vi "Main.vi"() -> ()   [LabVIEW 2015]
doc: "Use this template to build a master/slave design pattern. The master loop always executes. It notifies one or more slave loops to execute their code. The slave loop(s) continue executing until they complete, then wait for another notification. Contrast this with the Producer/Consumer pattern in which the consumer loops execute only when they have data in their queue."
uses:
  System SubVIs/Notifier Messages.ctl
panel:
  out "BPM Size":bool
  out "Axis Positions":sgl[](array[numeric])
  in  "Run Scan":bool
  in  "Home Motors":bool
  in  "stop":bool
  # "X1"
  # "Y1"
  # "X2"
  # "Y2"
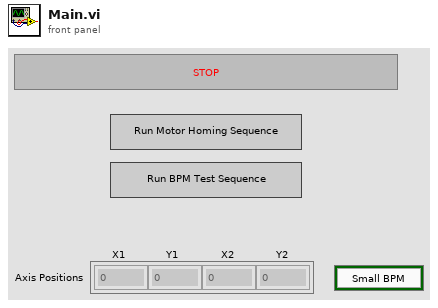
[diagram p1: front panel]
types:
  T1 = typedef "Notifier Messages.ctl" = enum16{"Do Nothing", "Run Scan", "Home Motors"}
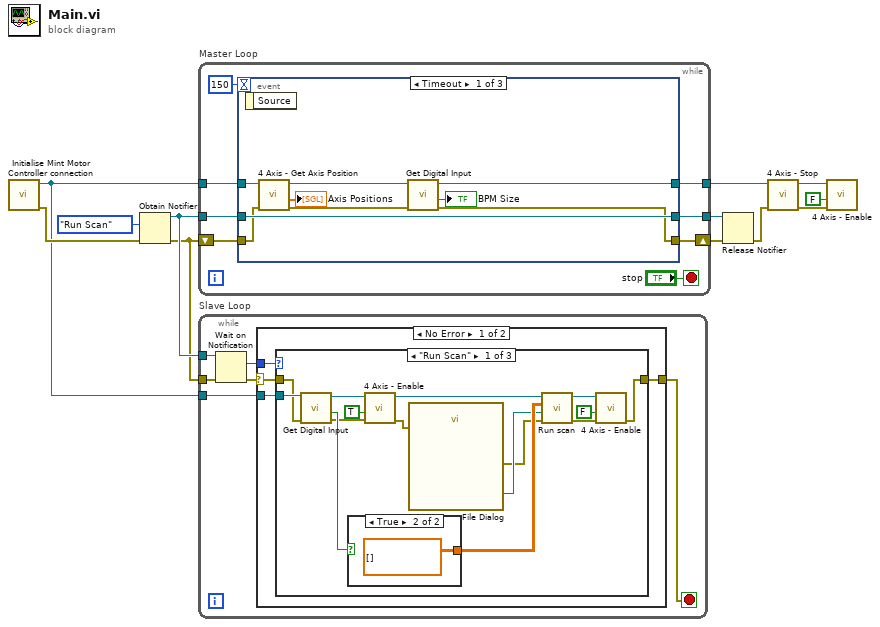
[diagram p0: block diagram]
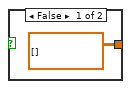
[diagram p2: hidden frame]
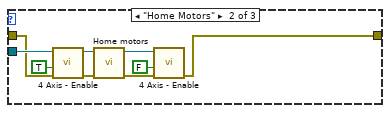
[diagram p3: hidden frame]
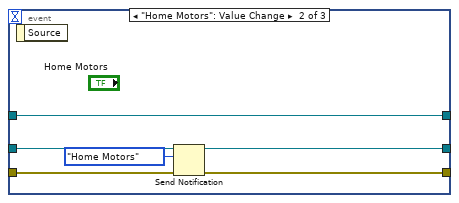
[diagram p6: hidden frame]
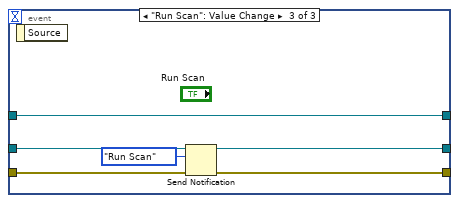
[diagram p7: hidden frame]
diagram:
  n1 = call "Initialise Mint Motor Controller connection.vi"() -> ("error out"=w7:errorcluster, "Controller reference out"=w6:refnum<k7>)  [unwired: 6 in]
  n2 = Obtain Notifier(notification data type=Notifier_Messages."Run Scan", error in (no error)=w7) -> (notifier out=w12:refnum<notifier>, error out=w8:errorcluster)  [unwired: 1 in, 2 out]
  n3 = while "Master Loop" {
    shift-right: [w15] -> w11
    shift-left: w8 -> [w17]
    tunnel: w12 -> [w18]
    tunnel: [w16] -> w10
    tunnel: w6 -> [w14]
    tunnel: [w13] -> w5
    stop <- "stop" stop-if-true
    n4 = event shown="[0] Timeout" {
      selector: _ -> [_ _ _]
      dyn-events: _ -> [_ _ _]
      timeout: 150 -> [_ _ _]
      tunnel: w18 -> [w29 w35 w41]
      tunnel: w17 -> [w27 w34 w40]
      tunnel: [w29 w33 w39] -> w16
      tunnel: [w23 w32 w38] -> w15
      tunnel: w14 -> [w28 w30 w36]
      tunnel: [w21 w30 w36] -> w13
      event Timeout {
        n5 = event-data() -> ()  [unwired: 1 in, 1 out]
        n6 = call "4 Axis - Get Axis Position.vi"("error in (no error)"=w27, "Controller Reference In"=w28) -> ("error out"=w25:errorcluster, "Axis Positions"=→"Axis Positions":sgl[], "Controller Reference Out"=w24:refnum<k7>)  [unwired: 3 in]
        n7 = call "Get Digital Input.vi"("error in (no error)"=w25, "Controller Reference"=w24) -> ("error out"=w23:errorcluster, "Boolean Value"=→"BPM Size":bool, "Controller Reference out"=w21:refnum<k7>)  [unwired: 2 in, 1 out]
      }
      event "Home Motors": Value Change {
        n8 = event-data() -> ()  [unwired: 1 in, 1 out]
        n9 = Send Notification(notification=Notifier_Messages."Home Motors", notifier=w35, error in (no error)=w34) -> (notifier out=w33:refnum<notifier>, error out=w32:errorcluster)
      }
      event "Run Scan": Value Change {
        n10 = event-data() -> ()  [unwired: 1 in, 1 out]
        n11 = Send Notification(notification=Notifier_Messages."Run Scan", notifier=w41, error in (no error)=w40) -> (notifier out=w39:refnum<notifier>, error out=w38:errorcluster)
      }
    }
  }
  n12 = while "Slave Loop" {
    tunnel: w12 -> [w47]
    tunnel: w8 -> [w44]
    tunnel: w6 -> [w43]
    stop <- w42 stop-if-true
    n13 = Wait on Notification(notifier=w47, error in (no error)=w44) -> (notification=w45:T1, error out=w46:errorcluster)  [unwired: 4 out]
    n14 = case shown="No Error" w46 {
      selector: w46 -> [w50 w79]
      tunnel: w45 -> [w51 _]
      tunnel: w43 -> [w49 _]
      tunnel: [w48 w79] -> w42
      frame No Error {
        n15 = case shown="\"Run Scan\"" w51 {
          tunnel: w50 -> [w62 w74 w78]
          tunnel: w49 -> [w63 w75 _]
          tunnel: [w54 w70 w78] -> w48
          frame "Run Scan" {
            n16 = call "Get Digital Input.vi"("error in (no error)"=w62, "Controller Reference"=w63) -> ("error out"=w59:errorcluster, "Boolean Value"=w61:bool, "Controller Reference out"=w60:refnum<k7>)  [unwired: 2 in, 1 out]
            n17 = case shown="True" w61 {
              tunnel: [sgl[][] [] ("Position List") sgl[][] [] ("Position List")] -> w66
              frame False {
              }
              frame True {
              }
            }
            n18 = call "4 Axis - Enable.vi"("error in (no error)"=w59, "Enable/Disable"=TRUE, "Controller Reference In"=w60) -> ("error out"=w57:errorcluster, "Controller Reference Out"=w56:refnum<k7>)  [unwired: 3 in]
            n19 = call "File Dialog"("error in"=w57) -> ("selected path"=w65:path, "error out"=w64:errorcluster)  [unwired: 11 in, 2 out]
            n20 = call "Run scan.vi"("error in (no error)"=w64, "Log file path"=w65, "Position List"=w66, "Controller Reference In"=w56) -> ("error out"=w55:errorcluster, "Controller Reference Out"=w53:refnum<k7>)  [unwired: 1 in, 1 out]
            n21 = call "4 Axis - Enable.vi"("error in (no error)"=w55, "Enable/Disable"=FALSE, "Controller Reference In"=w53) -> ("error out"=w54:errorcluster)  [unwired: 3 in, 1 out]
          }
          frame "Home Motors" {
            n22 = call "4 Axis - Enable.vi"("error in (no error)"=w74, "Enable/Disable"=TRUE, "Controller Reference In"=w75) -> ("error out"=w77:errorcluster, "Controller Reference Out"=w76:refnum<k7>)  [unwired: 3 in]
            n23 = call "Home motors.vi"("error in (no error)"=w77, "Controller Reference In"=w76) -> ("error out"=w72:errorcluster, "Controller Reference Out"=w71:refnum<k7>)  [unwired: 4 in]
            n24 = call "4 Axis - Enable.vi"("error in (no error)"=w72, "Enable/Disable"=FALSE, "Controller Reference In"=w71) -> ("error out"=w70:errorcluster)  [unwired: 3 in, 1 out]
          }
          frame "Do Nothing", Default {
          }
        }
      }
      frame Error {
      }
    }
  }
  n25 = Release Notifier(notifier=w10, error in (no error)=w11) -> (error out=w4:errorcluster)  [unwired: 3 out]
  n26 = call "4 Axis - Stop.vi"("error in (no error)"=w4, "Controller Reference"=w5) -> ("error out"=w3:errorcluster, "Controller Reference out"=w2:refnum<k7>)  [unwired: 4 in]
  n27 = call "4 Axis - Enable.vi"("error in (no error)"=w3, "Enable/Disable"=FALSE, "Controller Reference In"=w2) -> ()  [unwired: 3 in, 2 out]
